vi "System-EngineRunTime.vi"(1 "Loop Period [ms]":u32, 2 "DSI Reference":refnum<class "DCM-DSI.lvclass">) -> ()   [LabVIEW 2016, in "DSI-RT.lvlib"]
uses:
  DSI-RT.lvlib
  Classes/DCM-DSI/DCM-DSI.lvclass
  Classes/DCM-DSI/Read EPTx Data.vi
  <vilib>/Utility/config.llb/Read Key (U32).vi
  <vilib>/Utility/config.llb/Write Key (U32).vi
  <vilib>/addons/Software Calibration Management/xSCM/CalPoint.xnode
  <vilib>/Utility/config.llb/NI_LVConfig.lvlib
  <vilib>/addons/Software Calibration Management/xSCM/ni_scm.dll
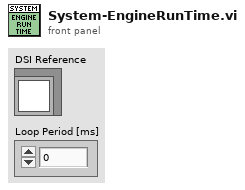
[diagram p1: front panel]
types:
  T1 = typedef "NI_LVConfig.lvlib/Config Data RefNum.ctl" = refnum<k1>
  T2 = typedef "EPTx - RevA - RT.lvlib/EPTxData.ctl" = cluster{"Sync":bool, "CurrentCAD":sgl, "Speed [RPM]":sgl, "Config":bool, "Rcvg Primary":bool, "Stall":bool, "Overflow":bool, "Ratio Error":bool, "Pattern Error":bool, "Aux Warning":bool, "Watchdog Error":bool}
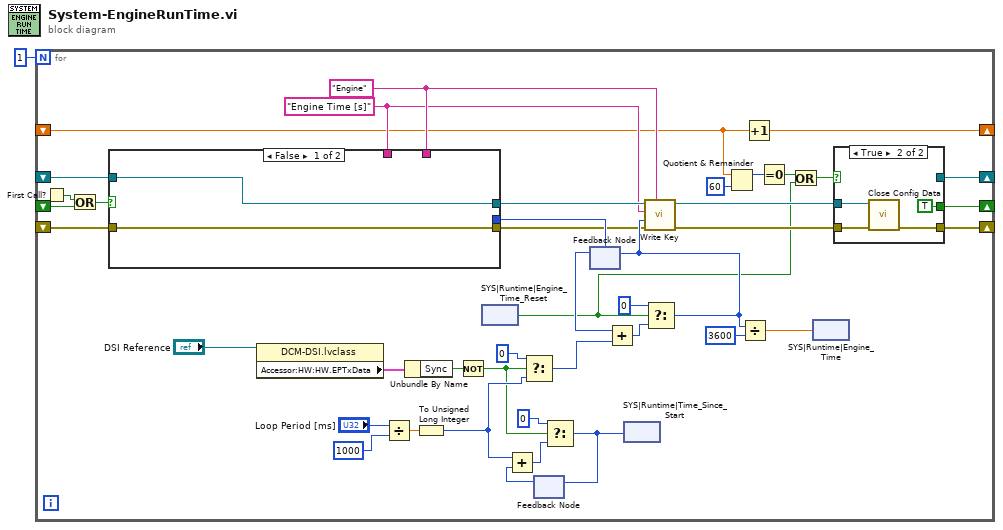
[diagram p0: block diagram]
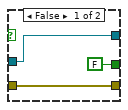
[diagram p2: hidden frame]
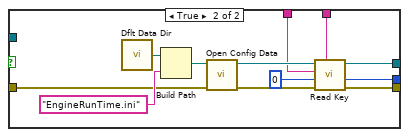
[diagram p3: hidden frame]
diagram:
  n1 = for {
    N: 1 -> [_]
    shift-right: [w22] -> _
    shift-left: _ -> [w11]
    shift-right: [w13] -> _
    shift-left: _ -> [w10]
    shift-right: [w9] -> _
    shift-left: _ -> [w8]
    shift-right: [w6] -> _
    shift-left: _ -> [w7]
    w17 = "Engine Time [s]" ("key")
    w18 = "Engine" ("section")
    n2 = First Call?() -> (First Call?: T/F=w12:bool)
    n3 = Or(x=w12, y=w11) -> (x .or. y?=w21:bool)
    n4 = case shown="False" w21 {
      tunnel: [_ w83] -> w28
      tunnel: [w71 w81] -> w20
      tunnel: w17 -> [_ w80]
      tunnel: w18 -> [_ w79]
      tunnel: [w72 w74] -> w15
      tunnel: w10 -> [w72 w73]
      tunnel: w8 -> [w71 _]
      frame False {
      }
      frame True {
        n5 = call <vilib>:"Dflt Data Dir.vi"() -> ("App:Default Data Directory"=w78:path)
        n6 = Build Path(base path=w78, name or relative path="EngineRunTime.ini" ("section")) -> (appended path=w76:path)
        n7 = call <vilib>:"Open Config Data.vi"("error in (no error)"=w73, "configuration file path"=w76) -> ("error out"=w75:errorcluster, "refnum"=w84:T1)  [unwired: 7 in, 1 out]
        n8 = call-poly <vilib>:"Read Key.vi"("section"=w79, "error in (no error)"=w75, "default value"=u32 0, "key"=w80, "refnum"=w84) -> ("error out"=w74:errorcluster, "value"=w83:u32, "refnum out"=w81:T1)  [unwired: 3 in, 1 out]
      }
    }
    n9 = property class="DCM-DSI.lvclass"(reference="DSI Reference") -> ("Accessor:HW:HW.EPTxData"=w4:T2)  [unwired: 1 in, 2 out]
    n10 = Divide(x="Loop Period [ms]", y=u32 1000) -> (x/y=w37:dbl)
    n11 = Unbundle By Name(w4) -> ("Sync"=w27:bool)
    n12 = To Unsigned Long Integer(number=w37) -> (unsigned 32bit integer=w30:u32)
    n13 = Not(x=w27) -> (.not. x?=w23:bool)
    n14 = xnode "SYS|Runtime|Engine_Time_Reset"() -> ("Value"=w2:bool)
    n15 = Select(t=u32 0, s=w23, f=w30) -> (s? t:f=w40:u32)
    n16 = feedback #1() -> (w33:u32)  [unwired: 1 in]
    n17 = Add(x=w30, y=w33) -> (x+y=w32:u32)
    n18 = Select(t=u32 0, s=w23, f=w32) -> (s? t:f=w34:u32)
    n19 = feedback-in #1(w34) -> ()
    n20 = feedback #2(w28) -> (w29:u32)
    n21 = Add(x=w29, y=w40) -> (x+y=w42:u32)
    n22 = xnode "SYS|Runtime|Time_Since_Start"("Value"=w34) -> ()
    n23 = Select(t=u32 0, s=w2, f=w42) -> (s? t:f=w16:u32)
    n24 = feedback-in #2(w16) -> ()
    n25 = call-poly <vilib>:"Write Key.vi"("section"=w18, "error in (no error)"=w15, "value"=w16, "key"=w17, "refnum"=w20) -> ("error out"=w14:errorcluster, "refnum out"=w19:T1)  [unwired: 4 in, 1 out]
    n26 = Quotient & Remainder(x=w7, y=u64 60) -> (x-y*floor(x/y)=w25:u64)  [unwired: 1 out]
    n27 = Divide(x=w16, y=u32 3600) -> (x/y=w35:dbl)
    n28 = Increment(x=w7) -> (x+1=w6:dbl)
    n29 = Equal To 0?(x=w25) -> (x = 0?=w24:bool)
    n30 = Or(x=w24, y=w2) -> (x .or. y?=w3:bool)
    n31 = xnode "SYS|Runtime|Engine_Time"("Value"=w35) -> ()
    n32 = case shown="True" w3 {
      tunnel: w19 -> [w64 w69]
      tunnel: [FALSE TRUE] -> w22
      tunnel: w14 -> [w65 w68]
      tunnel: [w65 w67] -> w13
      tunnel: [w64 _] -> w9
      frame False {
      }
      frame True {
        n33 = call <vilib>:"Close Config Data.vi"("error in (no error)"=w68, "refnum"=w69) -> ("error out"=w67:errorcluster)  [unwired: 8 in, 1 out]
      }
    }
  }
